vi "BRig_dataExp_T_ENL2_step.vi"() -> (2 "output_T_ENL2_step":i32)   [LabVIEW 2014]
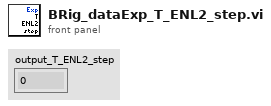
[diagram p1: front panel]
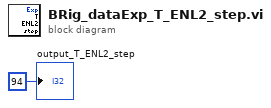
[diagram p0: block diagram]
diagram:
  "output_T_ENL2_step" <- 94 ("output_iBlock")
